vi "Wash Steps Selected.vi"(8 "error in (no error)":errorcluster, 11 "Wash Options Ref":refnum<vi>) -> (0 "error out":errorcluster, 1 "Wash Steps Selected-Update Display Message":T1)   [LabVIEW 2020]
doc: "This VI reads the Wash Options menu and creates an array with the selected options."
uses:
  Controls/Wash Steps Selected-Update Display Message.ctl
  Controls/Wash Steps Selected.ctl
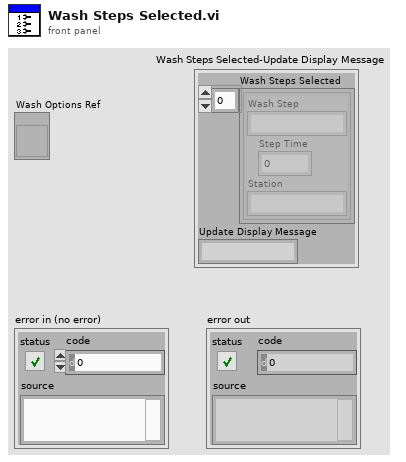
[diagram p1: front panel]
types:
  T1 = typedef "Wash Steps Selected-Update Display Message.ctl" = cluster{"Wash Steps Selected":cluster{"Wash Step":string, "Step Time":i32, "Station":string}[], "Update Display Message":string}
  T2 = enum8{"Enabled", "Disabled", "Disabled and Grayed Out"}
  T3 = cluster{bool, bool, bool, bool, bool, bool, bool, bool}
  T4 = typedef "Wash Steps Selected.ctl" = cluster{"Wash Step":string, "Step Time":i32, "Station":string}[]
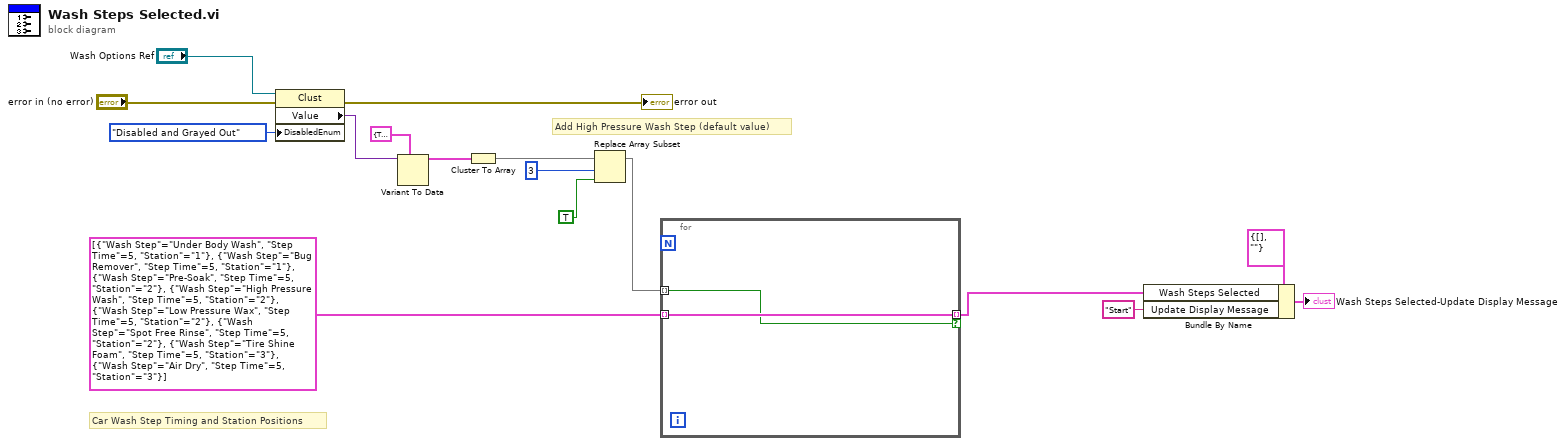
[diagram p0: block diagram]
diagram:
  # "Add High Pressure Wash Step (default value)"
  # "Car Wash Step Timing and Station Positions"
  n1 = property class="Clust"(reference="Wash Options Ref", error in="error in (no error)", "DisabledEnum"=T2."Disabled and Grayed Out" ("Disabled")) -> (error out=→"error out":errorcluster, "Value"=w13:variant)  [unwired: 1 out]
  n2 = Variant To Data(type=T3 {TRUE, TRUE, TRUE, TRUE, TRUE, TRUE, TRUE, TRUE}, Variant=w13) -> (data=w11:T3)  [unwired: 1 in, 1 out]
  n3 = Cluster To Array(cluster=w11) -> (array=w6:bool[])
  n4 = Replace Array Subset(array=w6, new element=TRUE ("new element/subarray"), index=3) -> (w3:bool[])
  n5 = for {
    tunnel: w3 -> [w17] mode=indexing
    tunnel: T4 [{"Wash Step"="Under Body Wash", "Step Time"=5, "Station"="1"}, {"Wash Step"="Bug Remover", "Step Time"=5, "Station"="1"}, {"Wash Step"="Pre-Soak", "Step Time"=5, "Station"="2"}, {"Wash Step"="High Pressure Wash", "Step Time"=5, "Station"="2"}, {"Wash Step"="Low Pressure Wax", "Step Time"=5, "Station"="2"}, {"Wash Step"="Spot Free Rinse", "Step Time"=5, "Station"="2"}, {"Wash Step"="Tire Shine Foam", "Step Time"=5, "Station"="3"}, {"Wash Step"="Air Dry", "Step Time"=5, "Station"="3"}] -> [w18] mode=indexing
    tunnel: [w18] -> w1 mode=indexing if=w17
  }
  n6 = Bundle By Name(cluster=T1 {"Wash Steps Selected"=[], "Update Display Message"=""}, "Wash Steps Selected"=w1, "Update Display Message"="Start") -> (→"Wash Steps Selected-Update Display Message":T1)
